vi "calibration_bounds.vi"(8 "Dynamixel Bounds":T1={"Main Dynamixel Set Data"={"Lower Winch Bound (deg)"=0.0, "Upper Winch Bound (deg)"=0.0}, "Rudder Dynamixel Set Data"={"Lower Winch Bound (deg)"=15.0, "Upper Winch Bound (deg)"=60.0}, "Jib Dynamixel Set Data"={"Lower Winch Bound (deg)"=0.0, "Upper Winch Bound (deg)"=0.0}}, 9 "Sail 2 Bound Offset":dbl=800.0, 10 "Sail 1 Bound Offset":dbl=800.0, 11 "VISA resource name in":refnum<visa-resource-name>) -> (3 "Dynamixel Bounds Out":T1)   [LabVIEW 2013]
doc: "This helper VI reads the current positions of the sail motors, and the lower bounds to those values.\n Its inputs are thecurrent bounds, which include the rudder bounds that are not set by the VI, and the sail bounds offsets, which are the difference between the upper and lower bounds.\n\nSean Carter\n11/12/14"
uses:
  Data/TypeDefs/MotorSetup.ctl
  Data/TypeDefs/DynamixelSetupInfo.ctl
  <instrlib>/Dynamixel Motor/Dynamixel Motor.lvlib
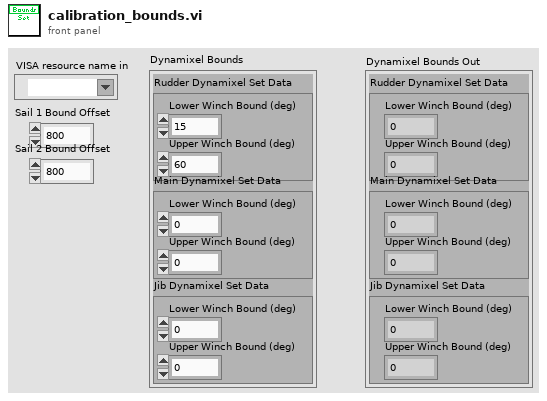
[diagram p1: front panel]
types:
  T1 = typedef "MotorSetup.ctl" = cluster{"Main Dynamixel Set Data":T2, "Rudder Dynamixel Set Data":T2, "Jib Dynamixel Set Data":T2}
  T2 = typedef "DynamixelSetupInfo.ctl" = cluster{"Lower Winch Bound (deg)":dbl, "Upper Winch Bound (deg)":dbl}
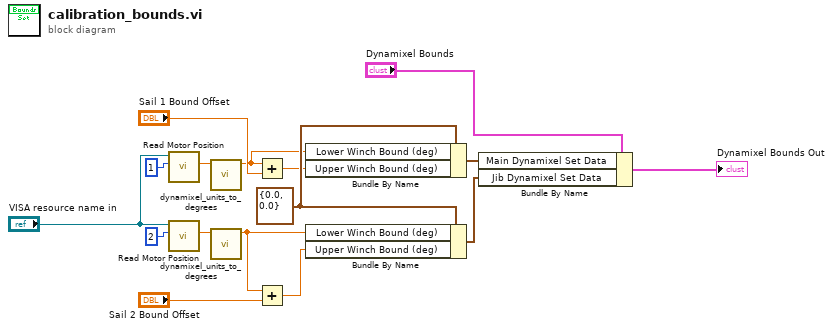
[diagram p0: block diagram]
diagram:
  w9 = T2 {"Lower Winch Bound (deg)"=0.0, "Upper Winch Bound (deg)"=0.0} ("Main Dynamixel Set Data")
  n1 = call <instrlib>:"Read Motor Position.vi"("Motor ID (0)"=u8 1, "VISA resource name"="VISA resource name in") -> ("Position (deg)"=w13:dbl)  [unwired: 7 in, 2 out]
  n2 = call <instrlib>:"Read Motor Position.vi"("Motor ID (0)"=u8 2, "VISA resource name"="VISA resource name in") -> ("Position (deg)"=w12:dbl)  [unwired: 7 in, 2 out]
  n3 = call "dynamixel_units_to_degrees.vi"("Dynamixel Input"=w13) -> ("Degrees"=w6:dbl)  [unwired: 9 in, 1 out]
  n4 = call "dynamixel_units_to_degrees.vi"("Dynamixel Input"=w12) -> ("Degrees"=w3:dbl)  [unwired: 9 in, 1 out]
  n5 = Add(x=w6, y="Sail 1 Bound Offset") -> (x+y=w5:dbl)
  n6 = Add(x=w3, y="Sail 2 Bound Offset") -> (x+y=w2:dbl)
  n7 = Bundle By Name(cluster=w9, "Lower Winch Bound (deg)"=w6, "Upper Winch Bound (deg)"=w5) -> (w11:T2)
  n8 = Bundle By Name(cluster=w9, "Lower Winch Bound (deg)"=w3, "Upper Winch Bound (deg)"=w2) -> (w10:T2)
  n9 = Bundle By Name(cluster="Dynamixel Bounds", "Main Dynamixel Set Data"=w11, "Jib Dynamixel Set Data"=w10) -> (→"Dynamixel Bounds Out":T1)
